vi "Write AutoCal Encrypted Password.vi"(8 "error in (no error)":errorcluster, 11 "Password":string) -> (0 "error out":errorcluster)   [LabVIEW 2015]
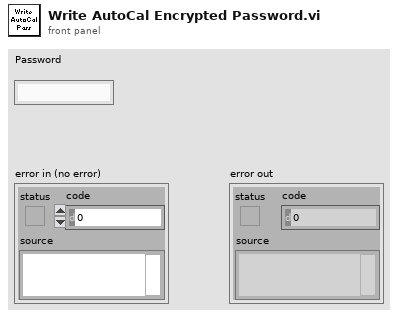
[diagram p1: front panel]
types:
  T1 = enum16{"open", "replace", "create", "open or create", "replace or create", "replace or create with confirmation"}
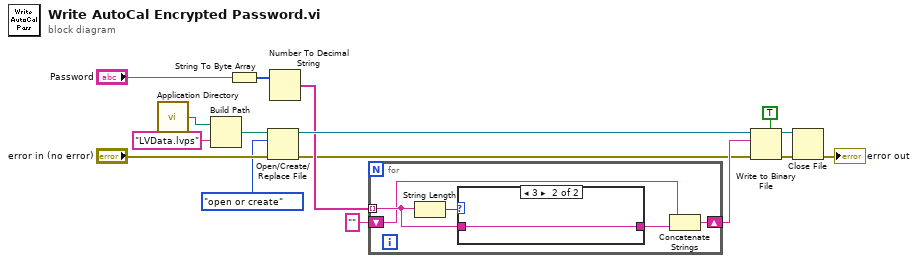
[diagram p0: block diagram]
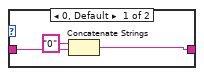
[diagram p2: hidden frame]
diagram:
  n1 = call <vilib>:"Application Directory.vi"() -> ("Application Directory"=w3:path)
  n2 = Build Path(base path=w3, name or relative path="LVData.lvps") -> (appended path=w1:path)
  n3 = String To Byte Array(string="Password") -> (unsigned byte array=w16:u8[])
  n4 = Open/Create/Replace File(file path (use dialog)=w1, error in="error in (no error)", operation (0:open)=T1."open or create") -> (refnum out=w12:refnum<file>, error out=w4:errorcluster)  [unwired: 3 in, 1 out]
  n5 = Number To Decimal String(number=w16) -> (decimal integer string=w9:string[])  [unwired: 1 in]
  n6 = for {
    tunnel: w9 -> [w20] mode=indexing
    shift-right: [w18] -> w6
    shift-left: "" -> [w17]
    n7 = String Length(string=w20) -> (length=w21:i32)
    n8 = case shown="3" w21 {
      tunnel: w20 -> [w23 w25]
      tunnel: [w22 w25] -> w19
      frame 0, Default {
        n9 = Concatenate Strings("0" ("string"), w23) -> (w22:string)
      }
      frame 3 {
      }
    }
    n10 = Concatenate Strings(w17, w19) -> (w18:string)
  }
  n11 = Write to Binary File(file (use dialog)=w12, data=w6, error in=w4, 5:TRUE ("prepend array or string size? (T)")) -> (refnum out=w15:refnum<file>, error out=w14:errorcluster)  [unwired: 2 in, 1 out]
  n12 = Close File(refnum=w15, error in=w14) -> (error out=→"error out":errorcluster)  [unwired: 1 out]
